vi "Rd Wr Filter Wheel Settings.vi"(7 "Wheel Name":string="Default", 8 "error in (no error)":errorcluster, 9 "Settings File":string="CC System Settings.json", 10 "Write? (F:Read)":bool, 11 "Filter Wheel Info":T1={"Num Wheels"=0, "Filters"=[], "Invalid Combinations"=[], "Addr"="", "Name"="", "Simulate"=FALSE, "Default Speed"=1000, "Homing"=[]} {"Default Speed" min=20 max=4000 step=10}) -> (0 "error out":errorcluster, 3 "Filter Wheel Settings":T1={"Num Wheels"=0, "Filters"=[], "Invalid Combinations"=[], "Addr"="", "Name"="", "Simulate"=FALSE, "Default Speed"=1000, "Homing"=[]} {"Default Speed" min=20 max=4000 step=10})   [LabVIEW 2024, in "Filter Wheel.lvclass"]
uses:
  Filter Wheel Object/Filter Wheel.lvclass
  Filter Wheel configuration.ctl
  Filter Wheel Object/Filter Wheel Details.ctl
  Filter Wheel Arduino Control/Filter Wheel Arduino Homing cluster.ctl
  65bd8ba7-6c5f-49c3-986f-02d69eb152e8.vi
  1ff77ff5-bc7f-48d0-940d-8d167d473090.vi
  <vilib>/JDP Science/JSONtext/Find Item.vi
  <vilib>/JDP Science/JSONtext/Next JSON Value.vi
  <vilib>/JDP Science/JSONtext/String Subset.vi
  <vilib>/JDP Science/JSONtext/Parsing/Advance past next JSON Value (inlined COPY).vi
  <vilib>/JDP Science/JSONtext/Parsing/Advance past whitespace.vi
  <vilib>/JDP Science/JSONtext/Parsing/Advance past String.vi
  <vilib>/JDP Science/JSONtext/Parsing/Advance past Number.vi
  <vilib>/JDP Science/JSONtext/Parsing/Advance past Line Ending.vi
  <vilib>/JDP Science/JSONtext/Parsing/Parse Full Path or Item Name.vi
  <vilib>/JDP Science/JSONtext/Parsing/Advance past Array.vi
  <vilib>/JDP Science/JSONtext/Parsing/Advance past Object.vi
  <vilib>/JDP Science/JSONtext/support/Error Cluster From Code.vi
  <vilib>/JDP Science/JSONtext/Offset/Find Item Locations by Path.vi
  <vilib>/JDP Science/JSONtext/JSON text to Variant.vi
  <vilib>/JDP Science/JSONtext/Variant to JSON Text.vi
  <vilib>/JDP Science/JSONtext/Set Item.vi
  <vilib>/JDP Science/JSONtext/LVClass Serializer/JSONtext LVClass Serializer.lvclass
  <vilib>/JDP Science/JSONtext/JSONtext.lvlib
panel:
  out "<JSON>":string caption="JSON"
  # "\"Filter Wheel Settings RIMAS\":{\n    \"Addr\":\"COM15\",\n    \"Default Speed\":200,\n    \"Filters\":[\n      {\n        \"Names\":[\"Grism\",\"Open\",\"Vph30\",\"Vph300\",\"Y\",\"J\"],\n        \"Relative Position\":[0,10000,17000,25000,33000,40000],\n        \"Size\":50000,\n        \"Wheel Name\":\"FW YJ\"\n      },\n      {\n        \"Names\":[\"Grism\",\"Open\",\"Vph30\",\"Vph300\",\"H\",\"K\"],\n        \"Relative Position\":[0,10000,17000,25000,33000,40000],\n        \"Size\":50000,\n        \"Wheel Name\":\"FW HK\"\n      },\n      {\n        \"Names\":[\n          \"K\",\n          \"Open\",\n          \"blank\",\n          \"Br-g\",\n          \"H2\",\n          \"2180\",\n          \"2190\"\n        ],\n        \"Relative Position\":[0,5560,11809,17908,23466,29016,34579],\n        \"Size\":40141,\n        \"Wheel Name\":\"Aux\"\n      },\n      {\n        \"Names\":[\n          \"blank\",\n          \"long\",\n          \"250 um\",\n          \"130 um\",\n          \"80 um\",\n          \"open\"\n        ],\n        \"Relative Position\":[0,5667,12889,20111,27333,34222],\n        \"Size\":40000,\n        \"Wheel Name\":\"Slit\"\n      }\n    ],\n    \"Homing Parameters\":{\n      \"Accel\":400,\n      \"Direction (F: CW)\":true,\n      \"Error Cnts\":300,\n      \"Homing Deltas\":[3000,3250,-680,-1560],\n      \"Speed\":400\n    },\n    \"Invalid Combinations\":[[]],\n    \"Name\":\"RIMAS\",\n    \"Num Wheels\":4,\n    \"Simulate\":false\n  },"
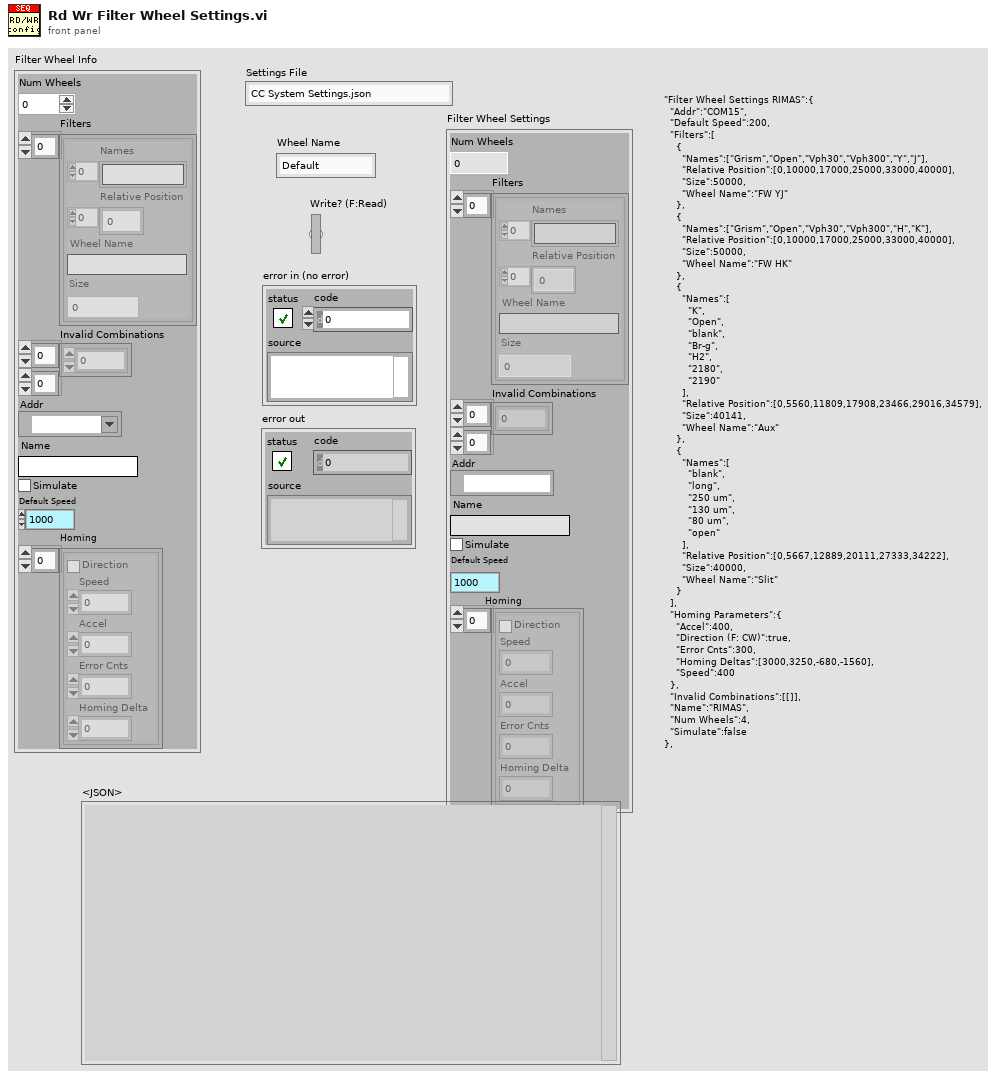
[diagram p1: front panel]
types:
  T1 = typedef "Filter Wheel.lvclass/Filter Wheel configuration.ctl" = cluster{"Num Wheels":i32, "Filters":T2[], "Invalid Combinations":i32[][], "Addr":refnum<visa-resource-name>, "Name":string, "Simulate":bool, "Default Speed":u16, "Homing":T3[]}
  T2 = typedef "Filter Wheel.lvclass/Filter Wheel Details.ctl" = cluster{"Names":string[], "Relative Position":i32[], "Wheel Name":string, "Size":i32}
  T3 = typedef "Filter Wheel Arduino Homing cluster.ctl" = cluster{"Direction":bool, "Speed":i32, "Accel":i32, "Error Cnts":i32, "Homing Delta":i32}
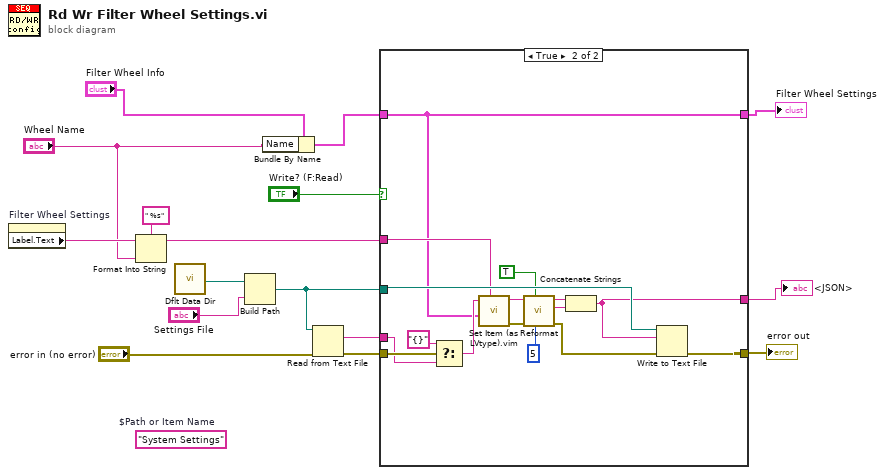
[diagram p0: block diagram]
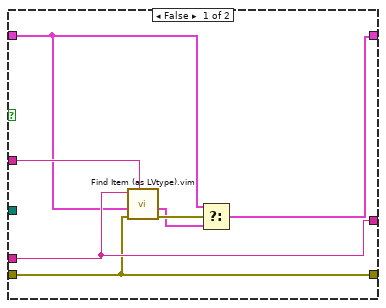
[diagram p2: hidden frame]
diagram:
  (unwired) "System Settings"  # $Path or Item Name
  n1 = property on="Filter Wheel Settings" class="Clust (strict)"() -> ("Label.Text"=w6:string)  [unwired: 2 in, 2 out]
  n2 = Format Into String(format string=" %s", initial string=w6, "Wheel Name") -> (resulting string=w4:string)  [unwired: 1 in, 1 out]
  n3 = call <vilib>:"Dflt Data Dir.vi"() -> ("App:Default Data Directory"=w16:path)
  n4 = Build Path(base path=w16, name or relative path="Settings File") -> (appended path=w12:path)
  n5 = Bundle By Name(cluster="Filter Wheel Info", "Name"="Wheel Name") -> (w5:T1)
  n6 = Read from Text File(file (use dialog)=w12, error in="error in (no error)") -> (text=w13:string, error out=w14:errorcluster)  [unwired: 2 in, 2 out]
  n7 = case shown="True" "Write? (F:Read)" {
    tunnel: w14 -> [w18 w36]
    tunnel: w5 -> [w19 w24]
    tunnel: w12 -> [_ w39]
    tunnel: [w18 w38] -> w11
    tunnel: [w17 w24] -> w2
    tunnel: w4 -> [w23 w37]
    tunnel: w13 -> [w20 w34]
    tunnel: [w20 w26] -> w8
    frame False {
      n8 = call "Find Item (as LVtype).vim"("$Path or Item Name"=w23, "error in (no error)"=w18, "Data Type and Default Value"=w19, "JSON"=w20) -> ("error out"=w22:errorcluster, "Data"=w21:T1)  [unwired: 4 in, 2 out]
      n9 = Select(t=w19, s=w22, f=w21) -> (s? t:f=w17:T1)
    }
    frame True {
      n10 = Select(t="{}" ("JSON"), s=w36, f=w34) -> (s? t:f=w33:string)
      n11 = call "Set Item (as LVtype).vim"("$Path or Item Name"=w37, "Anything"=w24, "JSON"=w33) -> ("error out"=w30:errorcluster, "<JSON>"=w31:string)  [unwired: 5 in, 1 out]
      n12 = call <vilib>:"Reformat.vi"("Pretty Print Levels"=5, "Alphabetically Sort Objects"=TRUE, "error in (no error)"=w30, "JSON"=w31) -> ("error out"=w29:errorcluster, "Rest of Input String"=w25:string, "<JSON>"=w28:string)  [unwired: 4 in, 1 out]
      n13 = Concatenate Strings(w28, w25) -> (w26:string)
      n14 = Write to Text File(file (use dialog)=w39, text=w26, error in=w29) -> (error out=w38:errorcluster)  [unwired: 1 in, 2 out]
    }
  }
  "error out" <- w11
  "Filter Wheel Settings" <- w2
  "<JSON>" <- w8
